vi "demo.vi"() -> ()   [LabVIEW 2024]
uses:
  Source/Interfaces/IRead Temperature/IRead Temperature.lvclass
  Source/Interfaces/IReadPressure/IRead Pressure.lvclass
  Source/Interfaces/IRead Dew Point/IRead Dew Point.lvclass
  Source/Interfaces/IRead Humidity/IRead Humidity.lvclass
  Source/Interfaces/IRead H2O Concentration/IRead H2O Concentration.lvclass
  Source/Interfaces/IRunnable/IRunnable.lvclass
  Source/Interfaces/IVirtual Instrument/IVirtual Instrument.lvclass
  Source/Instrument Manager/Instrument Manager.lvclass
panel:
  out "Error Out":errorcluster
  out "Temperature":dbl format="%.2f °C"
  out "Time Stamp t":timestamp format="%<%x %.3X>T"
  in  "stop":bool
  out "Pressure":dbl format="%d mbar a"
  out "Time Stamp p":timestamp format="%<%x %.3X>T"
  out "Dew Point":dbl format="%.2f °C"
  out "Time Stamp d":timestamp format="%<%x %.3X>T"
  out "iteration":i32
  out "Absolute Humidity":dbl format="%.1f g/m³"
  out "Time Stamp h":timestamp format="%<%x %.3X>T"
  out "H2O Concentration":dbl format="%d Vol.-%"
  out "Time Stamp c":timestamp format="%<%x %.3X>T"
  out "Supply Chart":T1(graph)
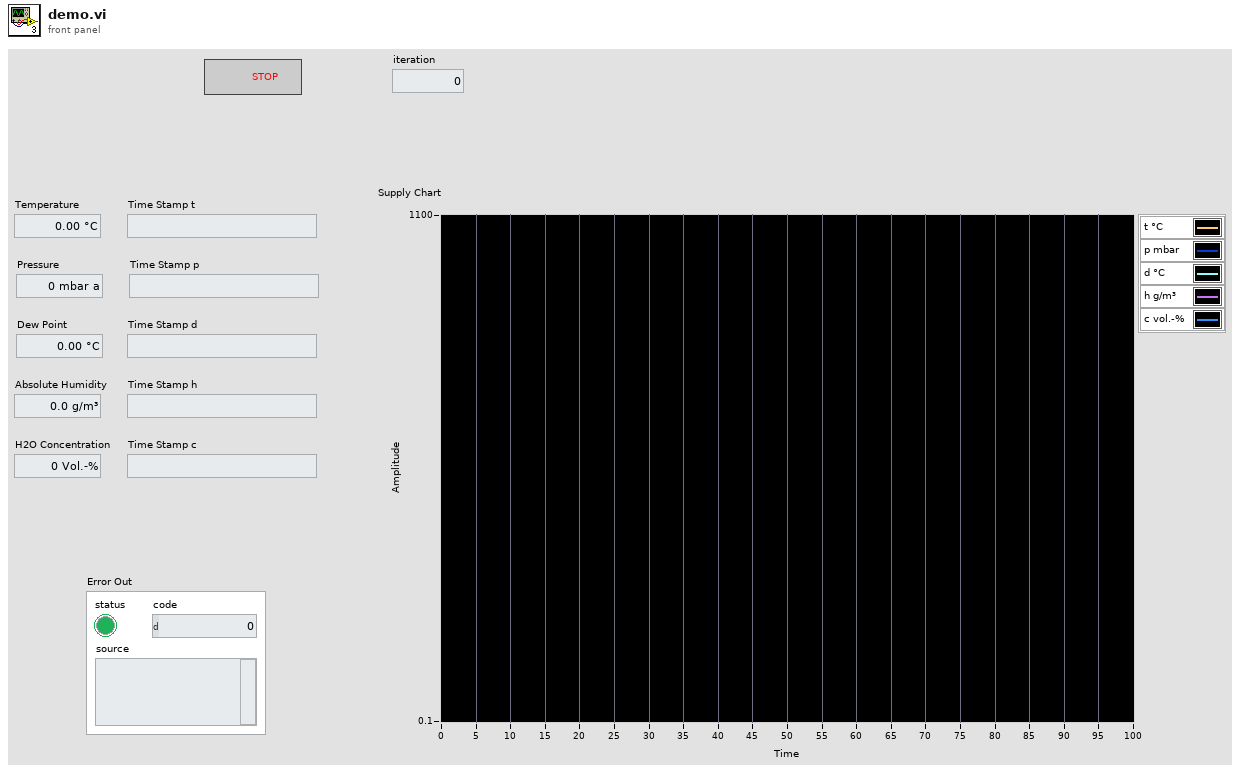
[diagram p1: front panel]
types:
  T1 = cluster{"Temperature":dbl, "Pressure":dbl, "Dew Point":dbl, "Humidity":dbl, "H2O Concentration":dbl}
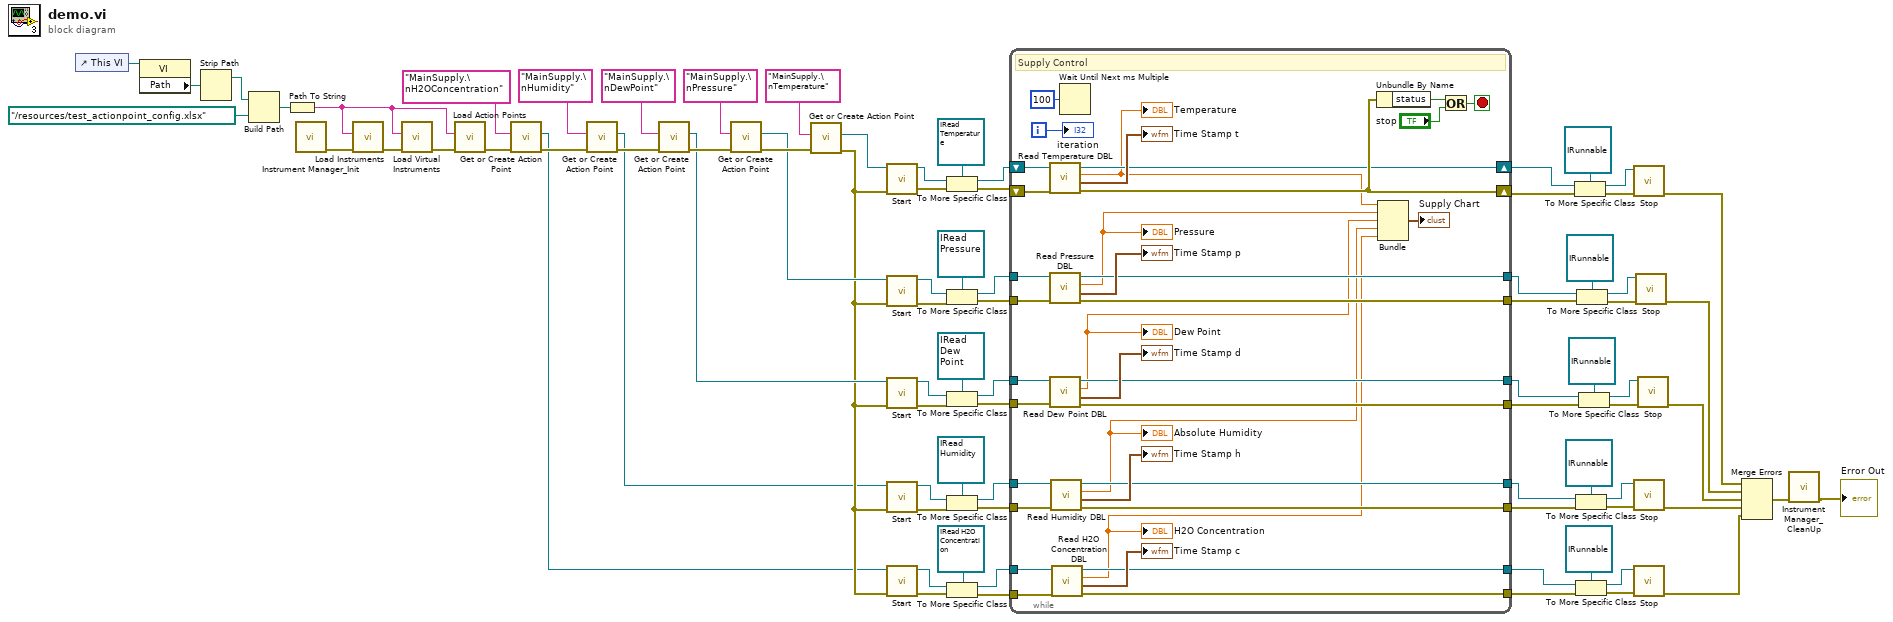
[diagram p0: block diagram]
diagram:
  n1 = control-ref of="This VI"() -> (w37:refnum<vi>)
  n2 = property class="VI"(reference=w37) -> ("Path"=w36:path)  [unwired: 1 in, 2 out]
  n3 = Strip Path(path=w36) -> (stripped path=w3:path)  [unwired: 1 out]
  n4 = Build Path(base path=w3, name or relative path=path "../resources/test_actionpoint_config.xlsx") -> (appended path=w4:path)
  n5 = Path To String(path=w4) -> (string=w2:string)
  n6 = call "Instrument Manager_Init.vi"() -> ("Error Out"=w81:errorcluster)  [unwired: 10 in, 1 out]
  n7 = call "Load Instruments.vi"("Error In"=w81, "Source"=w2) -> ("Error Out"=w79:errorcluster)  [unwired: 9 in]
  n8 = call "Load Virtual Instruments.vi"("Error In"=w79, "Source"=w2) -> ("Error Out"=w52:errorcluster)  [unwired: 9 in]
  n9 = call "Load Action Points.vi"("Error In"=w52, "Source"=w2) -> ("Error Out"=w6:errorcluster)  [unwired: 9 in]
  n10 = call "Get or Create Action Point.vi"("Error In"=w6, "Action Point Identifier"="MainSupply.\nH2OConcentration" ("Virtual Instrument Identifier")) -> ("Error Out"=w10:errorcluster, "IAction Point"=w7:refnum<class "IVirtual Instrument.lvclass">)  [unwired: 8 in]
  n11 = call "Get or Create Action Point.vi"("Error In"=w10, "Action Point Identifier"="MainSupply.\nHumidity" ("Virtual Instrument Identifier")) -> ("Error Out"=w19:errorcluster, "IAction Point"=w8:refnum<class "IVirtual Instrument.lvclass">)  [unwired: 8 in]
  n12 = call "Get or Create Action Point.vi"("Error In"=w19, "Action Point Identifier"="MainSupply.\nDewPoint" ("Instrument Identifier")) -> ("Error Out"=w51:errorcluster, "IAction Point"=w47:refnum<class "IVirtual Instrument.lvclass">)  [unwired: 8 in]
  n13 = call "Get or Create Action Point.vi"("Error In"=w51, "Action Point Identifier"="MainSupply.\nPressure" ("Virtual Instrument Identifier")) -> ("Error Out"=w78:errorcluster, "IAction Point"=w53:refnum<class "IVirtual Instrument.lvclass">)  [unwired: 8 in]
  n14 = call "Get or Create Action Point.vi"("Error In"=w78, "Action Point Identifier"="MainSupply.\nTemperature" ("Instrument Identifier")) -> ("Error Out"=w21:errorcluster, "IAction Point"=w38:refnum<class "IVirtual Instrument.lvclass">)  [unwired: 8 in]
  n15 = call-dynamic "Start.vi"("error in"=w21, "IRunnable in"=w38) -> ("error out"=w71:errorcluster, "IRunnable out"=w72:refnum<class "IVirtual Instrument.lvclass">)  [unwired: 8 in]
  n16 = call-dynamic "Start.vi"("error in"=w21, "IRunnable in"=w53) -> ("error out"=w68:errorcluster, "IRunnable out"=w67:refnum<class "IVirtual Instrument.lvclass">)  [unwired: 8 in]
  n17 = call-dynamic "Start.vi"("error in"=w21, "IRunnable in"=w47) -> ("error out"=w58:errorcluster, "IRunnable out"=w59:refnum<class "IVirtual Instrument.lvclass">)  [unwired: 8 in]
  n18 = call-dynamic "Start.vi"("error in"=w21, "IRunnable in"=w8) -> ("error out"=w34:errorcluster, "IRunnable out"=w33:refnum<class "IVirtual Instrument.lvclass">)  [unwired: 8 in]
  n19 = call-dynamic "Start.vi"("error in"=w21, "IRunnable in"=w7) -> ("error out"=w22:errorcluster, "IRunnable out"=w20:refnum<class "IVirtual Instrument.lvclass">)  [unwired: 8 in]
  n20 = To More Specific Class(target class=refnum<class "IRead Temperature.lvclass"> refnum ("IRead Temperature.lvclass"), reference=w72, error in=w71) -> (specific class reference=w69:refnum<class "IRead Temperature.lvclass">, error out=w70:errorcluster)
  n21 = To More Specific Class(target class=refnum<class "IRead Pressure.lvclass"> refnum ("IRead Pressure.lvclass"), reference=w67, error in=w68) -> (specific class reference=w55:refnum<class "IRead Pressure.lvclass">, error out=w54:errorcluster)
  n22 = To More Specific Class(target class=refnum<class "IRead Dew Point.lvclass"> refnum ("IRead Dew Point.lvclass"), reference=w59, error in=w58) -> (specific class reference=w56:refnum<class "IRead Dew Point.lvclass">, error out=w57:errorcluster)
  n23 = To More Specific Class(target class=refnum<class "IRead Humidity.lvclass"> refnum ("IRead Humidity.lvclass"), reference=w33, error in=w34) -> (specific class reference=w30:refnum<class "IRead Humidity.lvclass">, error out=w31:errorcluster)
  n24 = To More Specific Class(target class=refnum<class "IRead H2O Concentration.lvclass"> refnum ("IRead H2O Concentration.lvclass"), reference=w20, error in=w22) -> (specific class reference=w18:refnum<class "IRead H2O Concentration.lvclass">, error out=w23:errorcluster)
  n25 = while {
    shift-right: [w112] -> w76
    shift-left: w69 -> [w110]
    shift-right: [w113] -> w82
    shift-left: w70 -> [w111]
    tunnel: w57 -> [w107]
    tunnel: w56 -> [w106]
    tunnel: w55 -> [w105]
    tunnel: w54 -> [w104]
    tunnel: [w103] -> w40
    tunnel: [w102] -> w41
    tunnel: [w101] -> w42
    tunnel: [w100] -> w43
    tunnel: w31 -> [w98]
    tunnel: w30 -> [w97]
    tunnel: [w96] -> w29
    tunnel: [w94] -> w28
    tunnel: w23 -> [w93]
    tunnel: [w91] -> w13
    tunnel: w18 -> [w90]
    tunnel: [w89] -> w5
    i -> [w99]
    stop <- w116 stop-if-true
    # "Supply Control"
    n26 = call-dynamic "Read Temperature DBL.vi"("error in"=w111, "IRead Temperature in"=w110) -> ("error out"=w113:errorcluster, "Time Stamp"=→"Time Stamp t":timestamp, "Temperature"=w88:dbl, "IRead Temperature out"=w112:refnum<class "IRead Temperature.lvclass">)  [unwired: 6 in]
    "Temperature" <- w88
    n27 = call-dynamic "Read Pressure DBL.vi"("error in"=w104, "IRead Pressure in"=w105) -> ("error out"=w103:errorcluster, "Time Stamp"=→"Time Stamp p":timestamp, "Pressure"=w87:dbl, "IRead Pressure out"=w102:refnum<class "IRead Pressure.lvclass">)  [unwired: 6 in]
    "Pressure" <- w87
    n28 = call-dynamic "Read Dew Point DBL.vi"("error in"=w107, "IRead Dew Point in"=w106) -> ("error out"=w100:errorcluster, "Time Stamp"=→"Time Stamp d":timestamp, "Dew Point"=w86:dbl, "IRead Dew Point out"=w101:refnum<class "IRead Dew Point.lvclass">)  [unwired: 6 in]
    "Dew Point" <- w86
    n29 = call-dynamic "Read Humidity DBL.vi"("error in"=w98, "IRead Absolute Humidity in"=w97) -> ("error out"=w96:errorcluster, "Time Stamp"=→"Time Stamp h":timestamp, "Humidity"=w85:dbl, "IRead Absolute Humidity out"=w94:refnum<class "IRead Humidity.lvclass">)  [unwired: 6 in]
    "Absolute Humidity" <- w85
    n30 = call-dynamic "Read H2O Concentration DBL.vi"("error in"=w93, "IRead Water Concentration in"=w90) -> ("error out"=w91:errorcluster, "Time Stamp"=→"Time Stamp c":timestamp, "H2O Concentration"=w84:dbl, "IRead Water Concentration out"=w89:refnum<class "IRead H2O Concentration.lvclass">)  [unwired: 6 in]
    "H2O Concentration" <- w84
    n31 = Wait Until Next ms Multiple(millisecond multiple=u32 100) -> ()  [unwired: 1 out]
    n32 = Unbundle By Name(w113) -> ("status"=w114:bool)
    n33 = Bundle("Temperature"=w88, "Pressure"=w87, "Dew Point"=w86, "Humidity"=w85, "H2O Concentration"=w84) -> (→"Supply Chart":T1)  [unwired: 1 in]
    n34 = Or(x=w114, y="stop") -> (x .or. y?=w116:bool)
    "iteration" <- w99
  }
  n35 = To More Specific Class(target class=refnum<class "IRunnable.lvclass"> refnum ("IRunnable.lvclass"), reference=w76, error in=w82) -> (specific class reference=w74:refnum<class "IRunnable.lvclass">, error out=w77:errorcluster)
  n36 = To More Specific Class(target class=refnum<class "IRunnable.lvclass"> refnum ("IRunnable.lvclass"), reference=w28, error in=w29) -> (specific class reference=w25:refnum<class "IRunnable.lvclass">, error out=w27:errorcluster)
  n37 = To More Specific Class(target class=refnum<class "IRunnable.lvclass"> refnum ("IRunnable.lvclass"), reference=w5, error in=w13) -> (specific class reference=w15:refnum<class "IRunnable.lvclass">, error out=w14:errorcluster)
  n38 = To More Specific Class(target class=refnum<class "IRunnable.lvclass"> refnum ("IRunnable.lvclass"), reference=w41, error in=w40) -> (specific class reference=w65:refnum<class "IRunnable.lvclass">, error out=w63:errorcluster)
  n39 = To More Specific Class(target class=refnum<class "IRunnable.lvclass"> refnum ("IRunnable.lvclass"), reference=w42, error in=w43) -> (specific class reference=w44:refnum<class "IRunnable.lvclass">, error out=w46:errorcluster)
  n40 = call-dynamic "Stop.vi"("error in"=w77, "IRunnable in"=w74) -> ("error out"=w80:errorcluster)  [unwired: 8 in, 1 out]
  n41 = call-dynamic "Stop.vi"("error in"=w27, "IRunnable in"=w25) -> ("error out"=w26:errorcluster)  [unwired: 8 in, 1 out]
  n42 = call-dynamic "Stop.vi"("error in"=w14, "IRunnable in"=w15) -> ("error out"=w12:errorcluster)  [unwired: 8 in, 1 out]
  n43 = call-dynamic "Stop.vi"("error in"=w63, "IRunnable in"=w65) -> ("error out"=w61:errorcluster)  [unwired: 8 in, 1 out]
  n44 = call-dynamic "Stop.vi"("error in"=w46, "IRunnable in"=w44) -> ("error out"=w39:errorcluster)  [unwired: 8 in, 1 out]
  n45 = Merge Errors(w80, w61, w39, w26, w12) -> (w62:errorcluster)
  n46 = call "Instrument Manager_CleanUp.vi"("Error In"=w62) -> ("Error Out"=→"Error Out":errorcluster)  [unwired: 10 in]
